vi "Kill Session Management Service.vi"(8 "error in":errorcluster) -> (0 "error out":errorcluster)   [LabVIEW 2020, in "MeasurementServerTests.lvlib"]
uses:
  MeasurementServerTests.lvlib
  Runtime/APIs/Session Management V1/Session Reservation/Session Reservation.lvclass
  Runtime/APIs/Discovery V1/TypeDefs/gRPC Client Cache FGV Action.ctl
  Runtime/APIs/Discovery V1/Plug-In SDK Discovery V1 API.lvlib
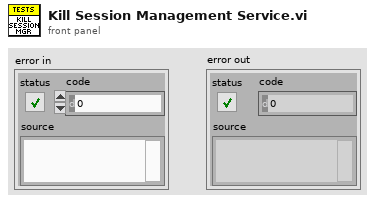
[diagram p1: front panel]
types:
  T1 = typedef "Plug-In SDK Discovery V1 API.lvlib/gRPC Client Cache FGV Action.ctl" = enum16{"Get Client", "Recreate Client", "Destroy Client", "Update ClusterId"}
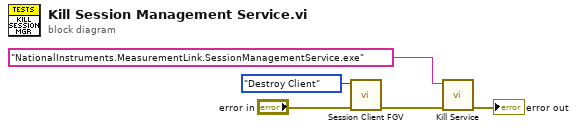
[diagram p0: block diagram]
diagram:
  n1 = call "Session Client FGV.vi"("error in"="error in", "action"=gRPC_Client_Cache_FGV_Action."Destroy Client") -> ("error out"=w3:errorcluster)  [unwired: 7 in, 2 out]
  n2 = call "Kill Service.vi"("error in"=w3, "full exe name"="NationalInstruments.MeasurementLink.SessionManagementService.exe" ("command line")) -> ("error out"=→"error out":errorcluster)  [unwired: 9 in]
